vi "RemapAENames.vi"(8 "error in (no error)":errorcluster, 9 "CISCO Agents":string[](array[string]), 10 "Current AE-NamesMapping":T1(array[cluster]), 11 "AE-NamesRaw (Repport)":string[](array[string])) -> (0 "error out":errorcluster)   [LabVIEW 2018, in "MainFrameLib.lvlib"]
uses:
  MainFrameLib.lvlib
panel:
  in  "Cancel":bool
  in  "Apply":bool
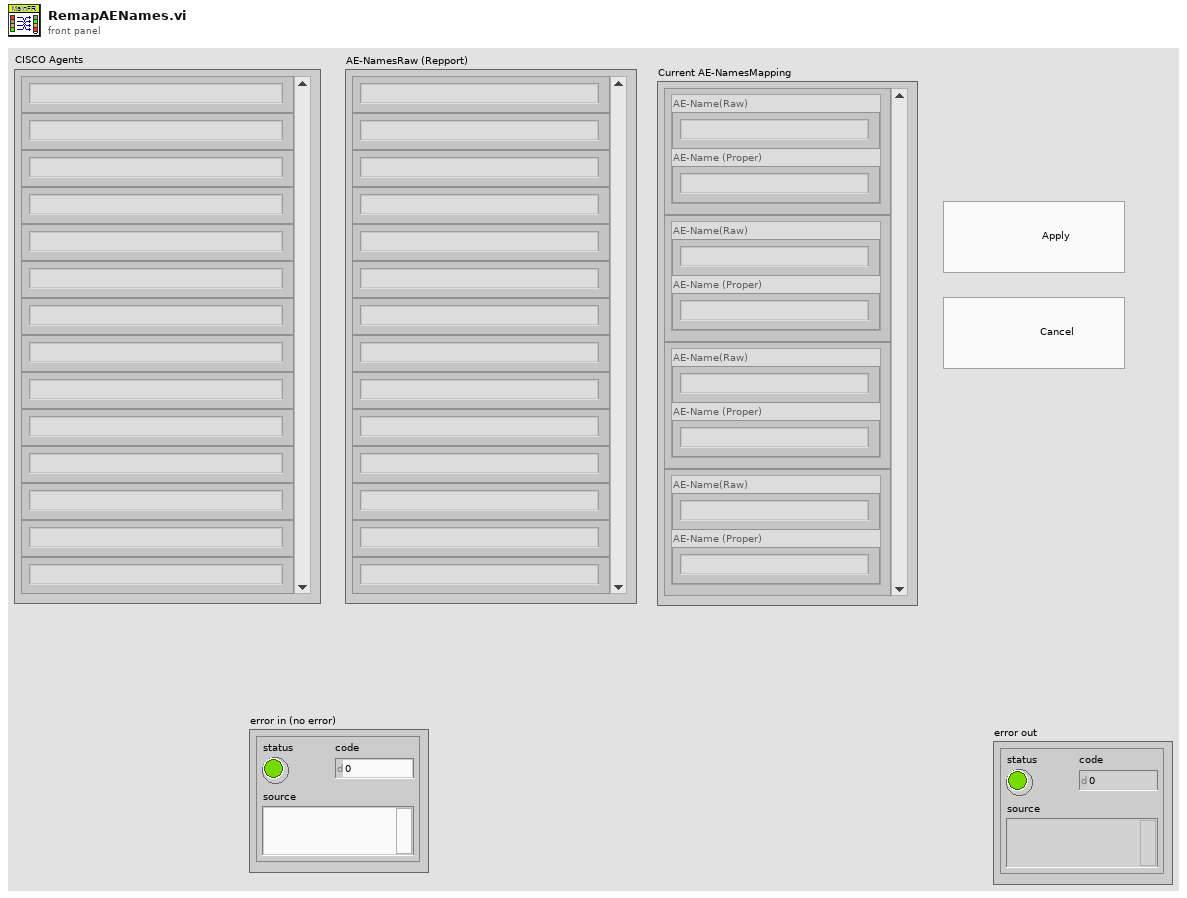
[diagram p1: front panel]
types:
  T1 = cluster{"AE-Name(Raw)":string, "AE-Name (Proper)":string}[]
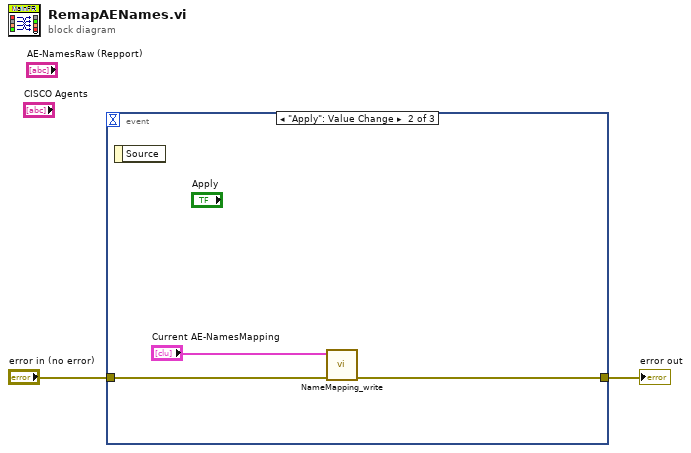
[diagram p0: block diagram]
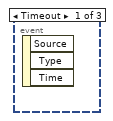
[diagram p2: hidden frame]
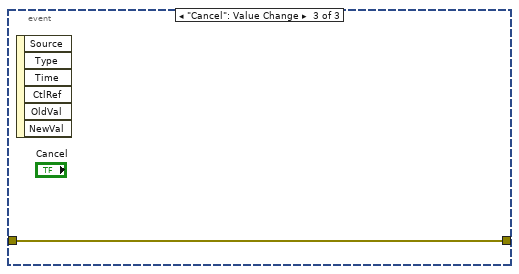
[diagram p3: hidden frame]
diagram:
  n1 = event shown="[1] \"Apply\": Value Change" {
    selector: _ -> [_ _ _]
    dyn-events: _ -> [_ _ _]
    timeout: _ -> [_ _ _]
    tunnel: "error in (no error)" -> [_ w5 w6]
    tunnel: [_ w3 w6] -> w1
    event Timeout {
      n2 = event-data() -> ()  [unwired: 1 in, 3 out]
    }
    event "Apply": Value Change {
      n3 = event-data() -> ()  [unwired: 1 in, 1 out]
      n4 = call "NameMapping_write.vi"("error in (no error)"=w5, "AE-NamesMapping"="Current AE-NamesMapping") -> ("error out"=w3:errorcluster)  [unwired: 9 in]
    }
    event "Cancel": Value Change {
      n5 = event-data() -> ()  [unwired: 1 in, 6 out]
    }
  }
  "error out" <- w1
